vi "Reset Osciloscope.vi"(8 "error in (no error)":errorcluster, 11 "OsciloscopeClass in":refnum<class "OsciloscopeClass.lvclass">) -> (0 "error out":errorcluster, 3 "OsciloscopeClass out":refnum<class "OsciloscopeClass.lvclass">)   [LabVIEW 2020, in "OsciloscopeClass.lvclass"]
uses:
  OsciloscopeClass.lvclass
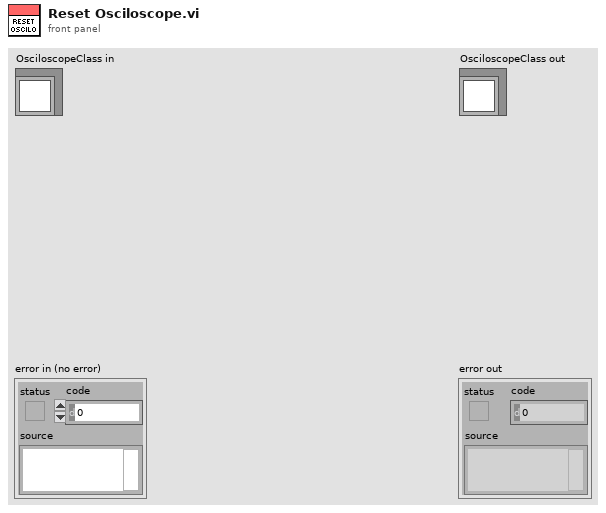
[diagram p1: front panel]
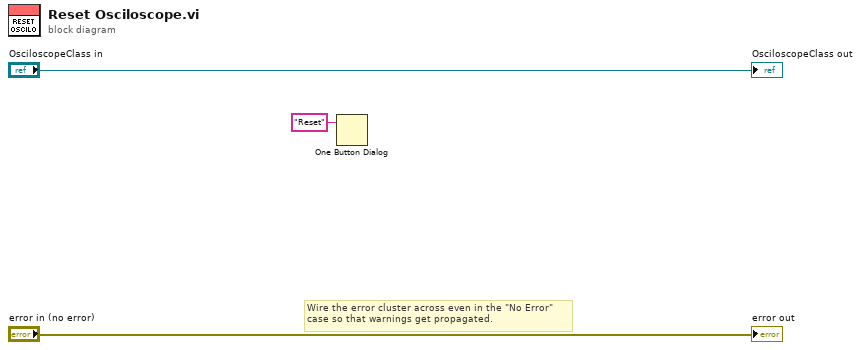
[diagram p0: block diagram]
diagram:
  # "Wire the error cluster across even in the \"No Error\"\ncase so that warnings get propagated."
  n1 = One Button Dialog(message="Reset") -> ()  [unwired: 1 in, 1 out]
  "error out" <- "error in (no error)"
  "OsciloscopeClass out" <- "OsciloscopeClass in"
